vi "Unflatten I64.vi"(3 "Flat Data":u8[](array[numeric]) format="%.0x", 4 "Endian":T1) -> (5 "I64":i64)   [LabVIEW 2021, in "DataTypes_CIF_U.lvlib"]
uses:
  DataTypes_CIF_U.lvlib
  Typedef/Endian.ctl
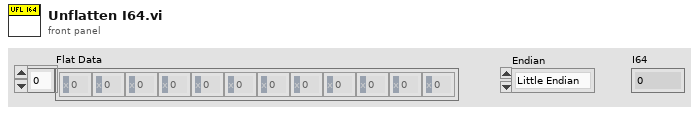
[diagram p1: front panel]
types:
  T1 = typedef "DataTypes_CIF_U.lvlib/Endian.ctl" = enum16{"Little Endian", "Big Endian"}
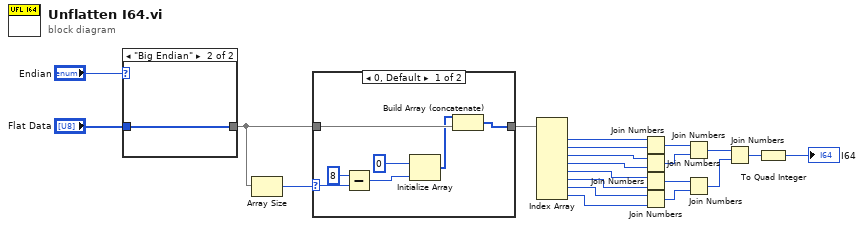
[diagram p0: block diagram]
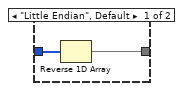
[diagram p3: hidden frame]
diagram:
  n1 = case shown="\"Big Endian\"" "Endian" {
    tunnel: "Flat Data" -> [w23 w24]
    tunnel: [w22 w24] -> w2
    frame "Little Endian", Default {
      n2 = Reverse 1D Array(array=w23) -> (reversed array=w22:u8[])
    }
    frame "Big Endian" {
    }
  }
  n3 = Array Size(array=w2) -> (size(s)=w5:i32)
  n4 = case shown="0, Default" w5 {
    selector: w5 -> [w31 _]
    tunnel: w2 -> [w27 w32]
    tunnel: [w25 w32] -> w3
    frame 0, Default {
      n5 = Subtract(x=8, y=w31) -> (x-y=w28:i32)
      n6 = Initialize Array(u8 0 ("element"), w28) -> (w26:u8[])
      n7 = Build Array (concatenate)(w26, w27) -> (w25:u8[])
    }
    frame 8.. {
    }
  }
  n8 = Index Array(array=w3) -> (element #1=w20:u8, element #2=w12:u8, element #3=w11:u8, element #4=w10:u8, element #5=w9:u8, element #6=w8:u8, element #7=w7:u8, element #8=w6:u8)  [unwired: 8 in]
  n9 = Join Numbers(hi=w20, lo=w12) -> ((hi.lo)=w19:u16)
  n10 = Join Numbers(hi=w11, lo=w10) -> ((hi.lo)=w14:u16)
  n11 = Join Numbers(hi=w9, lo=w8) -> ((hi.lo)=w17:u16)
  n12 = Join Numbers(hi=w7, lo=w6) -> ((hi.lo)=w13:u16)
  n13 = Join Numbers(hi=w19, lo=w14) -> ((hi.lo)=w18:u32)
  n14 = Join Numbers(hi=w17, lo=w13) -> ((hi.lo)=w16:u32)
  n15 = Join Numbers(hi=w18, lo=w16) -> ((hi.lo)=w15:u64)
  n16 = To Quad Integer(1:w15) -> (0:→"I64":i64)
